vi "Configure Trace Type.vi"(8 "error in (no error)":errorcluster, 10 "Trace Type (0: Clear Write)":u16(ring) items=["Clear Write", "Maximum Hold", "Minimum Hold", "View"], 11 "VISA resource name":refnum<visa-resource-name>) -> (0 "error out":errorcluster, 3 "VISA resource name out":refnum<visa-resource-name>)   [LabVIEW 2015, in "Template - Spectrum Analyzer.lvlib"]
doc: "Configures the type of trace to acquire."
uses:
  <instrlib>/_Template - Spectrum Analyzer/Template - Spectrum Analyzer.lvlib
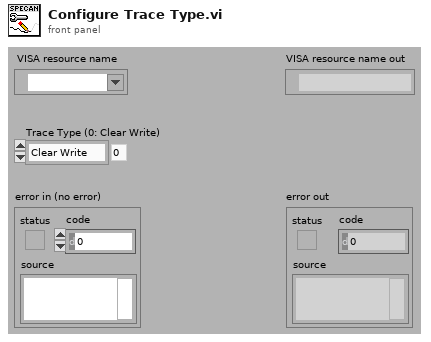
[diagram p1: front panel]
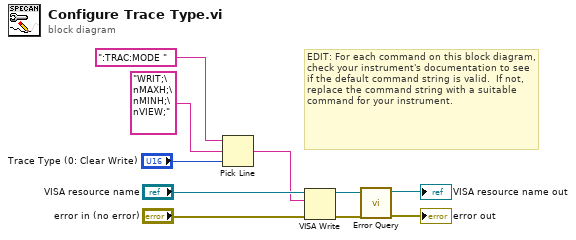
[diagram p0: block diagram]
diagram:
  # "EDIT: For each command on this block diagram, check your instrument's documentation to see if the default command string is valid.  If not, replace the command string with a suitable command for your instrument."
  n1 = Pick Line(string ("")=":TRAC:MODE ", multi-line string="WRIT;\nMAXH;\nMINH;\nVIEW;", line index="Trace Type (0: Clear Write)") -> (output string=w5:string)
  n2 = VISA Write(VISA resource name="VISA resource name", write buffer=w5, error in (no error)="error in (no error)") -> (VISA resource name out=w4:refnum<visa-resource-name>, error out=w2:errorcluster)  [unwired: 1 out]
  n3 = call <instrlib>:"Error Query.vi"("error in (no error)"=w2, "VISA resource name"=w4) -> ("error out"=→"error out":errorcluster, "VISA resource name out"=→"VISA resource name out":refnum<visa-resource-name>)  [unwired: 6 in, 2 out]
